vi "adc_samplepara.vi"(0 "channel_list":u8[](array[numeric])=[1], 5 "sample_mode":enum8{"序列采样", "分组采样", "同步采样"}(ring), 7 "frequency":u32, 9 "cycles":u32=1, 11 "group_interval":u32=1) -> (8 "adc_samplepara":T1={"channel_list "=[1], "channel_count"=0, "sample_mode"=0, "frequency"=0, "cycles"=1, "group_interval"=1})   [LabVIEW 2022 SP3, in "libdaqVI.lvlib"]
uses:
  libdaqVI.lvlib
panel:
  in  "adc_samplepara":T1={"channel_list "=[1], "channel_count"=0, "sample_mode"=0, "frequency"=0, "cycles"=1, "group_interval"=1}
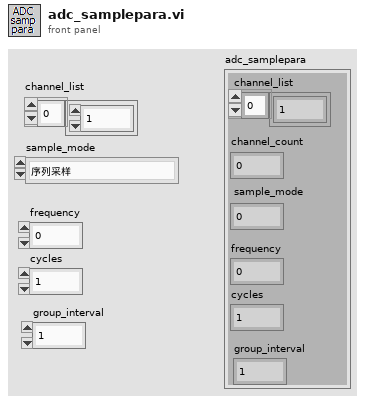
[diagram p1: front panel]
types:
  T1 = cluster{"channel_list ":u8[], "channel_count":u8, "sample_mode":u8, "frequency":u32, "cycles":u32, "group_interval":u32}
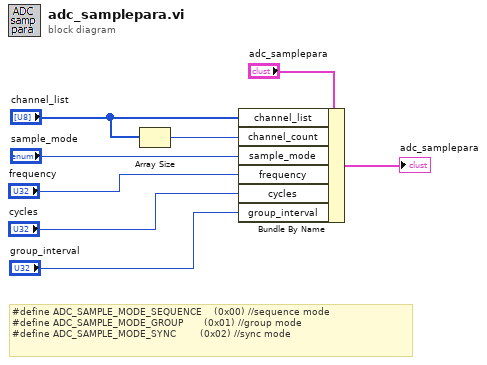
[diagram p0: block diagram]
diagram:
  # "#define ADC_SAMPLE_MODE_SEQUENCE    (0x00) //sequence mode\n#define ADC_SAMPLE_MODE_GROUP       (0x01) //group mode\n#define ADC_SAMPLE_MODE_SYNC        (0x02) //sync mode"
  n1 = Array Size(array="channel_list") -> (size(s)=w7:i32)
  n2 = Bundle By Name(cluster="adc_samplepara", "channel_list"="channel_list", "channel_count"=w7, "sample_mode"="sample_mode", "frequency"="frequency", "cycles"="cycles", "group_interval"="group_interval") -> (→"adc_samplepara":T1)
